vi "claustering trial 1.vi"() -> ()   [LabVIEW 2014]
panel:
  in  "List of common substrings and the number of times they occur":string[][](array[string])
  out "appended array 3":i32[](array[numeric])
  out "appended array 2":i32[](array[numeric])
  out "appended array":dbl[][][](array[numeric])
  in  "milliseconds to wait":u32
  out "3":string[](array[string])
  out "2":string[](array[string])
  out "1":string[](array[string])
  out "0":string[](array[string])
  out "Array":dbl[][](array[numeric])
  out "Weighted arrays 2":dbl[][][](array[numeric])
  out "Weighted arrays of cluster centers":dbl[][][](array[numeric])
  in  "Cluster centers":string[](array[string])=["-2 0 3 0 -3 0 4 -4 0\r\n", "0 3\r\n", "0 4 -3 0 -4 1 0 4 -3 0\r\n", "0\r\n", "-2 0 3 -3 0 -4 1 -4 0 3 -3 4 -3 0 2 0 3\r\n", "0 3 0 1\r\n", "0 1 0 3\r\n", "0 3 -2 0 4\r\n", "0\r\n", "0 -3 4 0 2 -2 0 -3 0 3 -2 3 -3 4\r\n", "0 -3 4 -3 0\r\n", "-2 0 -2 2 0\r\n", "0 3 -2\r\n", "0 4 -3 0 3 -2 0 -3 4 -3 0 3 -2 2 -2 0 4 0\r\n", "2 0 1 -4 0 3 0 -4 4 0 -4 4 0 2 0 4 0 -3 4 -3 0 -4 0 4\r\n", "0 4\r\n", "-2 0 -2 0 3 0\r\n", "0 3 0 -2 3\r\n", "0 4 0 4 -4 0 2 0 -4 4 -3 0 -2 2 -2 0 4 -3 0 2 0 3 0\r\n", "0 4 -3 0 1 -1 0 3 0 -2 2 -2 0 -3 4 -3 0 4 -4 1 0\r\n", "", "0 -3\r\n", "2 0 3 0 1 0 -2 3\r\n", "0\r\n", "1 -1 0\r\n", "0 -2 3 0\r\n", "0 1 0 4 0 4 -4 4\r\n", "0 1 -1 0 3\r\n", "0 2 -2 3 -3 4\r\n", "-2 2 0 -2 3\r\n", "0 -1\r\n", "0 4 -4 4 0 3 0 -2 0 -4 0 1 -4\r\n", "-2 0 4 0 -3 3 0 -2 2 -2 0 -4 0 4 0\r\n", "0 -1 0 -4 4 -4 1 -4 0\r\n", "1 -4 1 0 2 0 -3 0 2 0 -2 0 1 0 1 -4 4 -4 1 0 3 -2 0 -4 4 -4\r\n", "0 1 -4 4 -4 1\r\n", "0 3 0 -3 3 0 1 0 1 -4 4\r\n", "0 1 -4 0 1 -4\r\n", "0 3 -2 0 1 -4 1 0 2 0 4 0 4 0 -1 2 -1 0\r\n", "1 0 -1 0 2 0 4 -4\r\n", "-4\r\n", "-1 0 4\r\n", "0 1 -1 0 1 -4 0\r\n", "-1 0 1 -4 0 3 0 2 0 4 0 -4 4 -4 0 -1 0 -4 0 -2 0 4\r\n", "0 4 0\r\n", "0 4 -4 0 2 -1 0 2 0 4 -4 1 -4 4 0 3\r\n", "0 4 0 2 0\r\n", "1 0 -1 1 0 -4 1 -4 1 0 -4\r\n", "0 3 -2 0 -4\r\n", "2 -1 0 -4 4 -4 0 2 0 4\r\n", "1 0\r\n", "-1 0 -1 1 0 -4\r\n", "0 3 0\r\n", "0 -4 4 -4 0 -4 0 4 0 2 0 1 -4 4\r\n", "-1 0 1 -4\r\n", "-1 0 2 -1 0 2\r\n", "1 -1 0 4 -4 1\r\n", "-1 0 1 -4 4 -4 0 -4 4\r\n", "0 3 0 3 0 1 -1 0 1\r\n", "-1 0 4 0 4 -4 1 0 -4 0\r\n", "1 0 4\r\n", "0 -1 0 2 -1 0 -2 3 -2 0 -4 4 -4\r\n", "0 3 0\r\n", "2 -1 0 1 -4 4 -4 0 2 0\r\n", "0 4 -4 1 0 1 0 1 -4 0 2 0 4 0 4 -4 1\r\n", "1 -1 0 3 0 3 0 1 0 4\r\n", "0 -4 0 -2 0 -4\r\n", "0 -4 4 -4 0 -2 0 2 0\r\n", "-1 0 4 -4 0\r\n", "1 0 -1 2 0 4\r\n", "0 2 0 -2 0\r\n", "0 1 -4 0 -4 0 3 -2 0 -4 0 -4 4 -4 1\r\n", "0 4 0 4 0 4 0 4 0 -2 3 0 3 0 4 0\r\n", "-4 -1\r\n", "-2 0 1 0 -4 4\r\n", "0 4\r\n", "-2 2 0 -1 -4 1 0 3 0\r\n", "-1 0 -1 2\r\n", "0 -1 1 0 4 0 3 -2 0 -2 3 -2 0 4 0 -2 2\r\n", "2 -1 0 4\r\n", "0 4 0 2 0 -2 0\r\n", "1 -1 0 3 0 -4 4 -4 0\r\n", "2 -1 0 3 -2 0 -3 0 3 0 -3 0\r\n", "0 4 0 4 -4 1 -1 0 -3 0 1 -4 1 0 4 0 -4 0 -4 4 -4 1\r\n", "0 -4 1 0 -4 4\r\n", "0 4 0 -2 2 -2 2 -2 2\r\n", "-2 2 -1 0 4 0 2 0 4 0 2 -2 0 4\r\n", "1 0 -1 0 -1 0 1 -1\r\n", "-2 2 -2 3\r\n", "1 0 -1 0 -1 2 0 2 -2 0 -4 0\r\n", "-2 2 0 3 -2 2\r\n", "0\r\n", "1 -1 0 3\r\n", "0 4 0\r\n", "-2 0 1 -4 0 -3 0\r\n", "1 0 -1 2 -1 1 -4\r\n", "0 4\r\n", "-2 0 -1 1\r\n", "0 3 0 3 0 3 -2\r\n", "-4 0 -4 4\r\n", "0 4 0 -4 0 -4\r\n", "-2 2 0 4 -4 0 2 -2\r\n", "-2 2 -2 0 -1\r\n", "0 4 -3 0\r\n", "0 1 0 -1 1\r\n", "-4 0\r\n", "-2 0 3 0 1 0 3 -2 0 -1 0 4 0 3 0 -3 3 -3\r\n", "0 4 0 -2 0 1 0 -4 4 -3 0 1 0 4 0 -4 1 0 3 -3 0\r\n", "0 -1 2\r\n", "2 0 -3 4 0\r\n", "-4 0 -3 3 -3 0 -3 3 0 -2 3 0\r\n", "0 -1 1 -4 4 -3 0 3 0\r\n", "0 -1 2 0 3 0 1 -4 4 0 2 0\r\n", "2 -2 0 -4 0 -4 4 0 -4\r\n", "1 -1 2 -1\r\n", "2 0 -2 0 4 0 2 0 3 0 -2 0 -4\r\n", "1 -1 0 -1\r\n", "0 1 -4 1\r\n", "0 4 0 -1 1 -1 0\r\n", "0 3\r\n", "-2 0\r\n", "1 -4 0 -2 0 4 0 -4 0 4 -3 0 1 -4 0 1\r\n", "0 -3 3 -2 0 3 0 -2 2\r\n", "1 0\r\n", "2\r\n", "0 -4\r\n", "0 4 0 -4 0 -3 3 -3 0 -2 0 -2 0 4 0 -1 1 0 3 0 -4 1 -4 0 4\r\n", "2 0 -1 1\r\n", "0 2 0 4 0 4 -4 0 -1 2\r\n", "0 3 -2 0 3 -2\r\n", "1 0 -3 3 0 -4\r\n", "0 -3 3 0 -1 0\r\n", "2 -2 0 1\r\n", "-4 1 -4 1 -4 0\r\n", "0 4 0 2 0 -4 1 2 -1 0 4 0 1 0 4 -4 4 0 -4 4 0\r\n", "-2 0 3 0 -2 0\r\n"]
  in  "Full transition sequence from service to end":string[](array[string])=["-2 0 3 0 -3 0 4 -4 0\r\n", "0 3\r\n", "0 4 -3 0 -4 1 0 4 -3 0\r\n", "0\r\n", "-2 0 3 -3 0 -4 1 -4 0 3 -3 4 -3 0 2 0 3\r\n", "0 3 0 1\r\n", "0 1 0 3\r\n", "0 3 -2 0 4\r\n", "0\r\n", "0 -3 4 0 2 -2 0 -3 0 3 -2 3 -3 4\r\n", "0 -3 4 -3 0\r\n", "-2 0 -2 2 0\r\n", "0 3 -2\r\n", "0 4 -3 0 3 -2 0 -3 4 -3 0 3 -2 2 -2 0 4 0\r\n", "2 0 1 -4 0 3 0 -4 4 0 -4 4 0 2 0 4 0 -3 4 -3 0 -4 0 4\r\n", "0 4\r\n", "-2 0 -2 0 3 0\r\n", "0 3 0 -2 3\r\n", "0 4 0 4 -4 0 2 0 -4 4 -3 0 -2 2 -2 0 4 -3 0 2 0 3 0\r\n", "0 4 -3 0 1 -1 0 3 0 -2 2 -2 0 -3 4 -3 0 4 -4 1 0\r\n", "", "0 -3\r\n", "2 0 3 0 1 0 -2 3\r\n", "0\r\n", "1 -1 0\r\n", "0 -2 3 0\r\n", "0 1 0 4 0 4 -4 4\r\n", "0 1 -1 0 3\r\n", "0 2 -2 3 -3 4\r\n", "-2 2 0 -2 3\r\n", "0 -1\r\n", "0 4 -4 4 0 3 0 -2 0 -4 0 1 -4\r\n", "-2 0 4 0 -3 3 0 -2 2 -2 0 -4 0 4 0\r\n", "0 -1 0 -4 4 -4 1 -4 0\r\n", "1 -4 1 0 2 0 -3 0 2 0 -2 0 1 0 1 -4 4 -4 1 0 3 -2 0 -4 4 -4\r\n", "0 1 -4 4 -4 1\r\n", "0 3 0 -3 3 0 1 0 1 -4 4\r\n", "0 1 -4 0 1 -4\r\n", "0 3 -2 0 1 -4 1 0 2 0 4 0 4 0 -1 2 -1 0\r\n", "1 0 -1 0 2 0 4 -4\r\n", "-4\r\n", "-1 0 4\r\n", "0 1 -1 0 1 -4 0\r\n", "-1 0 1 -4 0 3 0 2 0 4 0 -4 4 -4 0 -1 0 -4 0 -2 0 4\r\n", "0 4 0\r\n", "0 4 -4 0 2 -1 0 2 0 4 -4 1 -4 4 0 3\r\n", "0 4 0 2 0\r\n", "1 0 -1 1 0 -4 1 -4 1 0 -4\r\n", "0 3 -2 0 -4\r\n", "2 -1 0 -4 4 -4 0 2 0 4\r\n", "1 0\r\n", "-1 0 -1 1 0 -4\r\n", "0 3 0\r\n", "0 -4 4 -4 0 -4 0 4 0 2 0 1 -4 4\r\n", "-1 0 1 -4\r\n", "-1 0 2 -1 0 2\r\n", "1 -1 0 4 -4 1\r\n", "-1 0 1 -4 4 -4 0 -4 4\r\n", "0 3 0 3 0 1 -1 0 1\r\n", "-1 0 4 0 4 -4 1 0 -4 0\r\n", "1 0 4\r\n", "0 -1 0 2 -1 0 -2 3 -2 0 -4 4 -4\r\n", "0 3 0\r\n", "2 -1 0 1 -4 4 -4 0 2 0\r\n", "0 4 -4 1 0 1 0 1 -4 0 2 0 4 0 4 -4 1\r\n", "1 -1 0 3 0 3 0 1 0 4\r\n", "0 -4 0 -2 0 -4\r\n", "0 -4 4 -4 0 -2 0 2 0\r\n", "-1 0 4 -4 0\r\n", "1 0 -1 2 0 4\r\n", "0 2 0 -2 0\r\n", "0 1 -4 0 -4 0 3 -2 0 -4 0 -4 4 -4 1\r\n", "0 4 0 4 0 4 0 4 0 -2 3 0 3 0 4 0\r\n", "-4 -1\r\n", "-2 0 1 0 -4 4\r\n", "0 4\r\n", "-2 2 0 -1 -4 1 0 3 0\r\n", "-1 0 -1 2\r\n", "0 -1 1 0 4 0 3 -2 0 -2 3 -2 0 4 0 -2 2\r\n", "2 -1 0 4\r\n", "0 4 0 2 0 -2 0\r\n", "1 -1 0 3 0 -4 4 -4 0\r\n", "2 -1 0 3 -2 0 -3 0 3 0 -3 0\r\n", "0 4 0 4 -4 1 -1 0 -3 0 1 -4 1 0 4 0 -4 0 -4 4 -4 1\r\n", "0 -4 1 0 -4 4\r\n", "0 4 0 -2 2 -2 2 -2 2\r\n", "-2 2 -1 0 4 0 2 0 4 0 2 -2 0 4\r\n", "1 0 -1 0 -1 0 1 -1\r\n", "-2 2 -2 3\r\n", "1 0 -1 0 -1 2 0 2 -2 0 -4 0\r\n", "-2 2 0 3 -2 2\r\n", "0\r\n", "1 -1 0 3\r\n", "0 4 0\r\n", "-2 0 1 -4 0 -3 0\r\n", "1 0 -1 2 -1 1 -4\r\n", "0 4\r\n", "-2 0 -1 1\r\n", "0 3 0 3 0 3 -2\r\n", "-4 0 -4 4\r\n", "0 4 0 -4 0 -4\r\n", "-2 2 0 4 -4 0 2 -2\r\n", "-2 2 -2 0 -1\r\n", "0 4 -3 0\r\n", "0 1 0 -1 1\r\n", "-4 0\r\n", "-2 0 3 0 1 0 3 -2 0 -1 0 4 0 3 0 -3 3 -3\r\n", "0 4 0 -2 0 1 0 -4 4 -3 0 1 0 4 0 -4 1 0 3 -3 0\r\n", "0 -1 2\r\n", "2 0 -3 4 0\r\n", "-4 0 -3 3 -3 0 -3 3 0 -2 3 0\r\n", "0 -1 1 -4 4 -3 0 3 0\r\n", "0 -1 2 0 3 0 1 -4 4 0 2 0\r\n", "2 -2 0 -4 0 -4 4 0 -4\r\n", "1 -1 2 -1\r\n", "2 0 -2 0 4 0 2 0 3 0 -2 0 -4\r\n", "1 -1 0 -1\r\n", "0 1 -4 1\r\n", "0 4 0 -1 1 -1 0\r\n", "0 3\r\n", "-2 0\r\n", "1 -4 0 -2 0 4 0 -4 0 4 -3 0 1 -4 0 1\r\n", "0 -3 3 -2 0 3 0 -2 2\r\n", "1 0\r\n", "2\r\n", "0 -4\r\n", "0 4 0 -4 0 -3 3 -3 0 -2 0 -2 0 4 0 -1 1 0 3 0 -4 1 -4 0 4\r\n", "2 0 -1 1\r\n", "0 2 0 4 0 4 -4 0 -1 2\r\n", "0 3 -2 0 3 -2\r\n", "1 0 -3 3 0 -4\r\n", "0 -3 3 0 -1 0\r\n", "2 -2 0 1\r\n", "-4 1 -4 1 -4 0\r\n", "0 4 0 2 0 -4 1 2 -1 0 4 0 1 0 4 -4 4 0 -4 4 0\r\n", "-2 0 3 0 -2 0\r\n"]
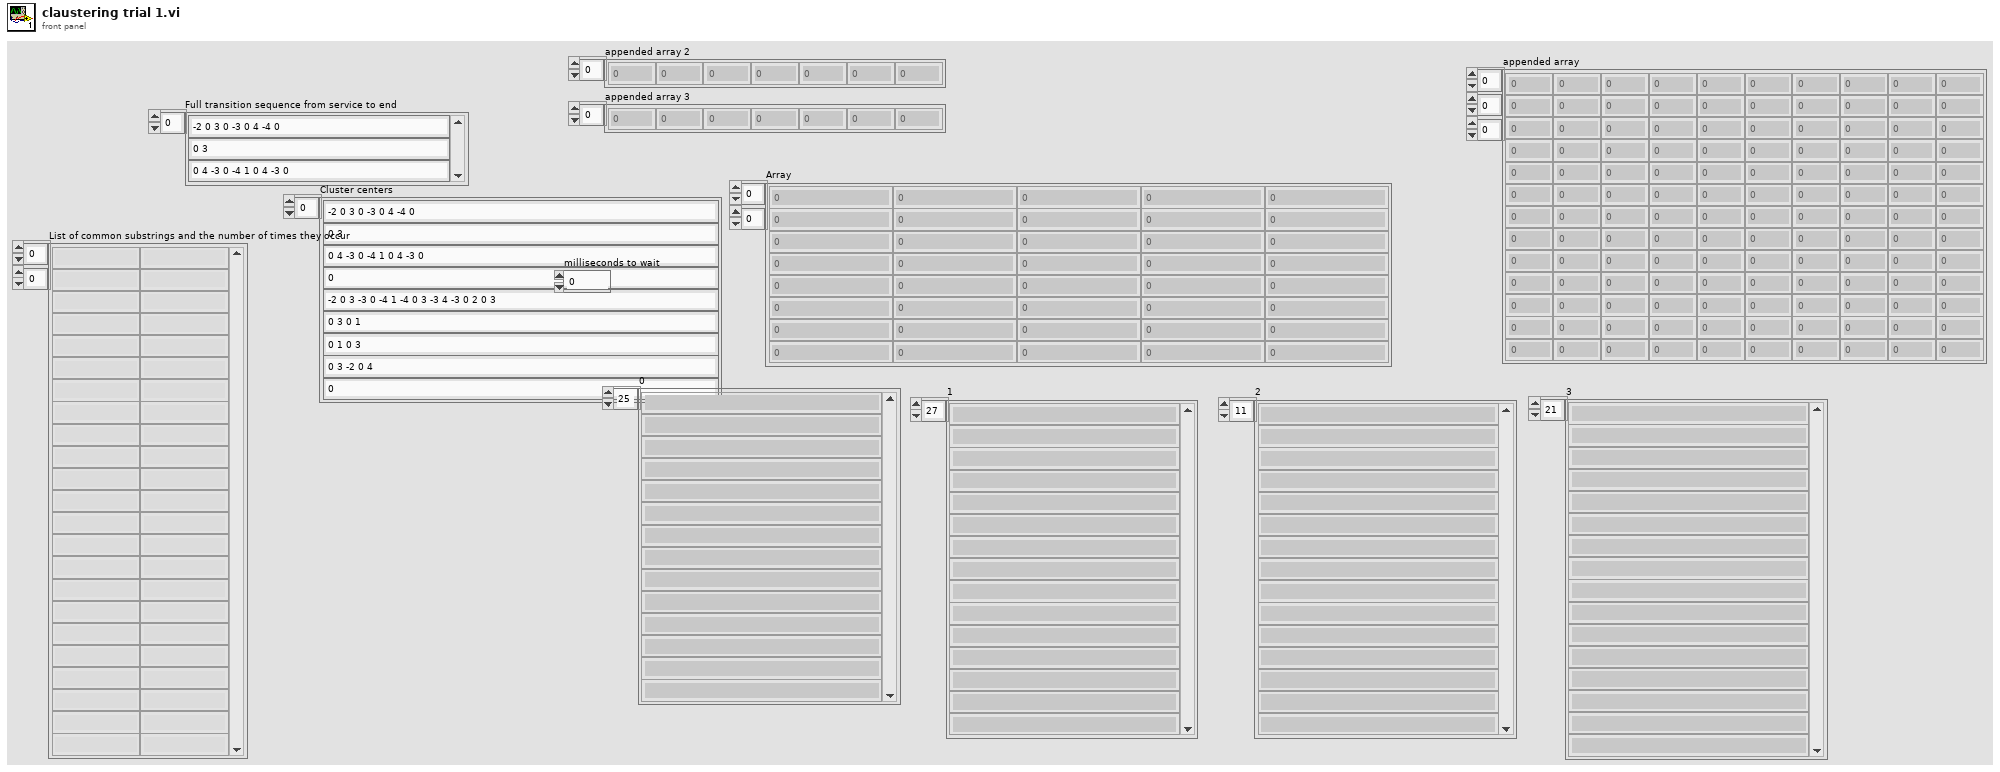
[diagram p1: front panel]
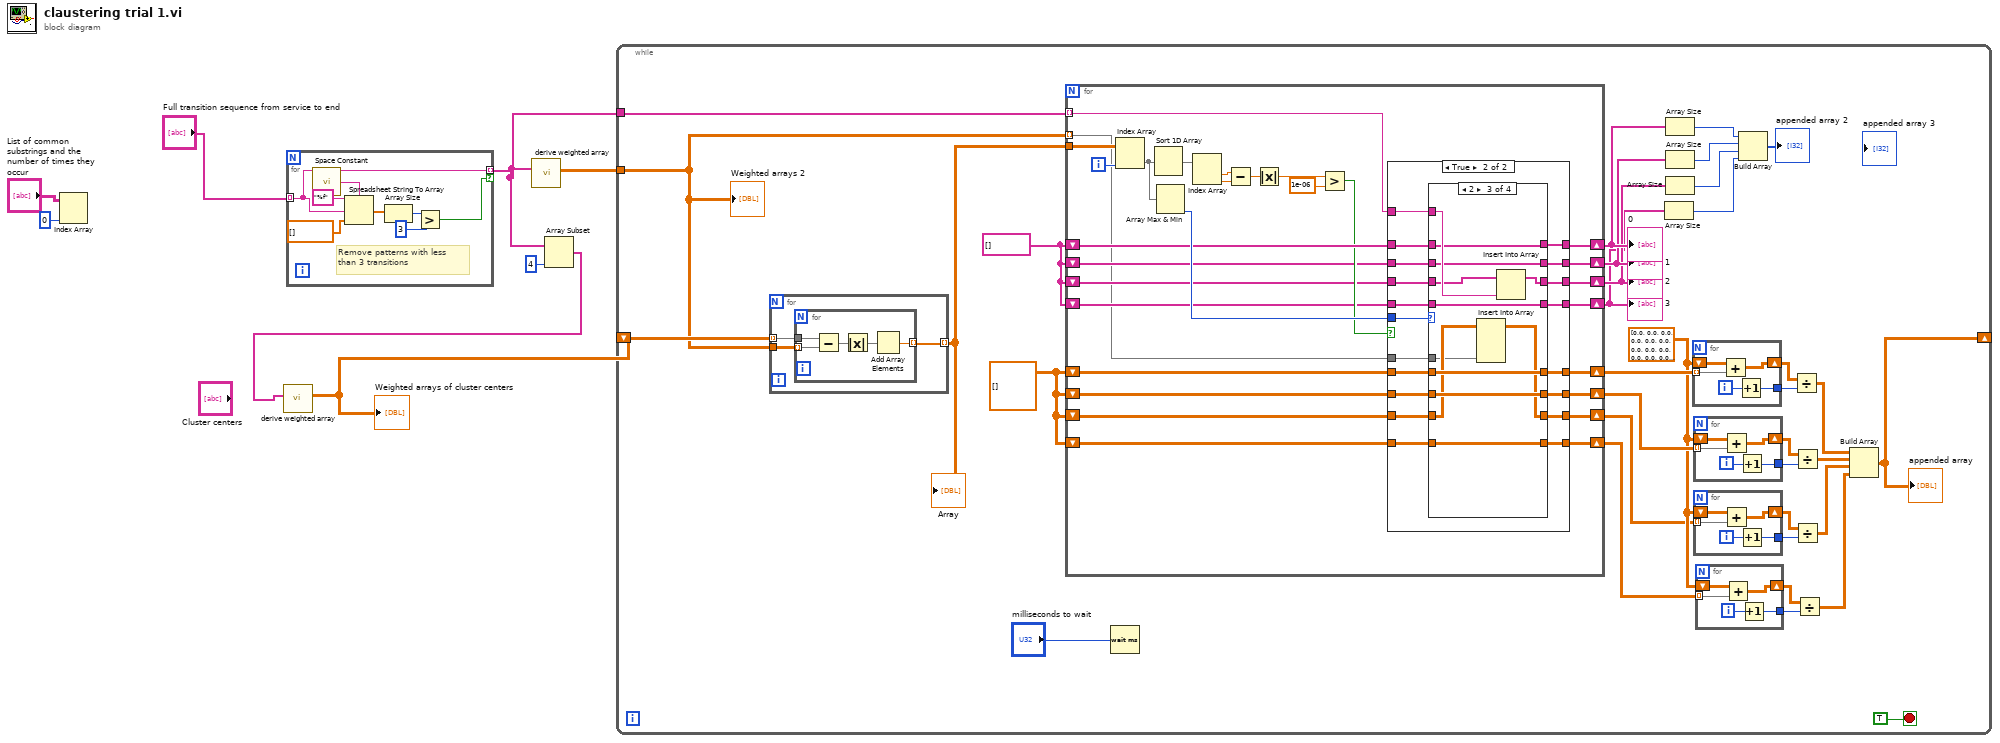
[diagram p0: block diagram]
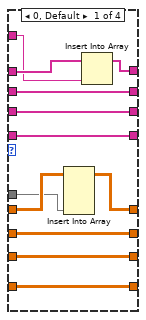
[diagram p3: hidden frame]
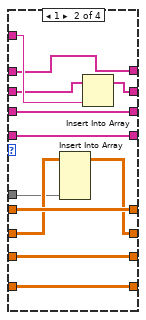
[diagram p4: hidden frame]
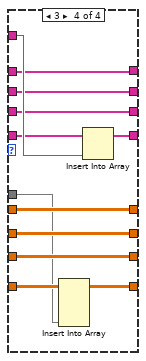
[diagram p5: hidden frame]
diagram:
  n1 = Index Array(array="List of common substrings and the number of times they occur", index (col)=0 ("disabled index (col)")) -> ()  [unwired: 1 in, 1 out]
  n2 = for {
    tunnel: "Full transition sequence from service to end" -> [w10] mode=indexing
    tunnel: [w10] -> w4 mode=indexing if=w9
    # "Remove patterns with less \nthan 3 transitions"
    n3 = call <vilib>:"Space Constant.vi"() -> ("String"=w15:string)
    n4 = Spreadsheet String To Array(delimiter (Tab)=w15, format string="%f", spreadsheet string=w10, array type (2D Dbl)=dbl[] [] ("array 2")) -> (array=w13:dbl[])
    n5 = Array Size(array=w13) -> (size(s)=w12:i32)
    n6 = Greater?(x=w12, y=3) -> (0:w9:bool)
  }
  n7 = call "derive weighted array.vi"("Full transition sequence from service to end"=w4) -> ("Weighted arrays"=w1:dbl[][][])  [unwired: 10 in]
  n8 = Array Subset(array=w4, length=4) -> (w3:string[])  [unwired: 1 in]
  n9 = call "derive weighted array.vi"("Full transition sequence from service to end"=w3) -> ("Weighted arrays"=w2:dbl[][][])  [unwired: 10 in]
  "Weighted arrays of cluster centers" <- w2
  n10 = while {
    tunnel: w4 -> [w49]
    shift-right: [w26] -> _
    shift-left: w2 -> [w51]
    tunnel: w1 -> [w50]
    stop <- TRUE stop-if-true
    w35 = dbl[][] [[0.0, 0.0, 0.0, 0.0, 0.0], [0.0, 0.0, 0.0, 0.0, 0.0], [0.0, 0.0, 0.0, 0.0, 0.0], [0.0, 0.0, 0.0, 0.0, 0.0], [0.0, 0.0, 0.0, 0.0, 0.0]] ("Weighted arrays")
    w46 = dbl[][][] [] ("Weighted arrays")
    w47 = string[] [] ("Full transition sequence from service to end")
    n11 = for {
      tunnel: w51 -> [w178] mode=indexing
      tunnel: w50 -> [w177]
      tunnel: [w176] -> w48 mode=indexing
      n12 = for {
        tunnel: w178 -> [w183]
        tunnel: w177 -> [w182] mode=indexing
        tunnel: [w179] -> w176 mode=indexing
        n13 = Subtract(x=w183, y=w182) -> (x-y=w181:dbl[][])
        n14 = Absolute Value(x=w181) -> (abs(x)=w180:dbl[][])
        n15 = Add Array Elements(numeric array=w180) -> (sum=w179:dbl)
      }
    }
    "Array" <- w48
    n16 = for {
      tunnel: w49 -> [w89] mode=indexing
      tunnel: w50 -> [w80] mode=indexing
      tunnel: w48 -> [w100]
      shift-right: [w88] -> w25
      shift-left: w47 -> [w90]
      shift-right: [w86] -> w24
      shift-left: w47 -> [w83]
      shift-right: [w85] -> w23
      shift-left: w47 -> [w82]
      shift-right: [w84] -> w22
      shift-left: w47 -> [w81]
      shift-right: [w79] -> w45
      shift-left: w46 -> [w78]
      shift-right: [w74] -> w36
      shift-left: w46 -> [w77]
      shift-right: [w73] -> w34
      shift-left: w46 -> [w76]
      shift-right: [w72] -> w33
      shift-left: w46 -> [w75]
      i -> [w93]
      n17 = Index Array(array=w100, index (col)=w93) -> (element=w92:dbl[])  [unwired: 1 in]
      n18 = Sort 1D Array(array=w92) -> (sorted array=w95:dbl[])
      n19 = Array Max & Min(array=w92) -> (min index (indices)=w91:i32)  [unwired: 3 out]
      n20 = Index Array(array=w95) -> (element #1=w99:dbl, element #2=w94:dbl)  [unwired: 2 in]
      n21 = Subtract(x=w99, y=w94) -> (x-y=w97:dbl)
      n22 = Absolute Value(x=w97) -> (abs(x)=w96:dbl)
      n23 = Greater?(x=w96, y=1e-06) -> (0:w87:bool)
      n24 = case shown="True" w87 {
        tunnel: w91 -> [_ w127]
        tunnel: w90 -> [w108 w126]
        tunnel: w89 -> [_ w125]
        tunnel: [w108 w124] -> w88
        tunnel: [w107 w120] -> w86
        tunnel: [w106 w119] -> w85
        tunnel: [w105 w118] -> w84
        tunnel: w83 -> [w107 w123]
        tunnel: w82 -> [w106 w122]
        tunnel: w81 -> [w105 w121]
        tunnel: w80 -> [_ w117]
        tunnel: [w104 w115] -> w79
        tunnel: w78 -> [w104 w116]
        tunnel: w77 -> [w103 w114]
        tunnel: w76 -> [w102 w113]
        tunnel: w75 -> [w101 w112]
        tunnel: [w103 w111] -> w74
        tunnel: [w102 w110] -> w73
        tunnel: [w101 w109] -> w72
        frame False {
        }
        frame True {
          n25 = case shown="2" w127 {
            tunnel: w126 -> [w139 w146 w161 w174]
            tunnel: w125 -> [w138 w151 w163 w175]
            tunnel: [w137 w146 w161 w174] -> w124
            tunnel: w123 -> [w136 w147 w158 w173]
            tunnel: w122 -> [w135 w150 w159 w170]
            tunnel: w121 -> [w134 w149 w162 w171]
            tunnel: [w136 w148 w158 w173] -> w120
            tunnel: [w135 w150 w160 w170] -> w119
            tunnel: [w134 w149 w162 w172] -> w118
            tunnel: w117 -> [w132 w141 w153 w165]
            tunnel: w116 -> [w133 w145 w157 w169]
            tunnel: [w131 w145 w157 w169] -> w115
            tunnel: w114 -> [w130 w142 w156 w168]
            tunnel: w113 -> [w129 w144 w154 w167]
            tunnel: w112 -> [w128 w143 w155 w166]
            tunnel: [w130 w140 w156 w168] -> w111
            tunnel: [w129 w144 w152 w167] -> w110
            tunnel: [w128 w143 w155 w164] -> w109
            frame 0, Default {
              n26 = Insert Into Array(array=w133, new element=w132) -> (w131:dbl[][][])  [unwired: 3 in]
              n27 = Insert Into Array(array=w139, new element=w138) -> (w137:string[])  [unwired: 1 in]
            }
            frame 1 {
              n28 = Insert Into Array(array=w142, new element=w141) -> (w140:dbl[][][])  [unwired: 3 in]
              n29 = Insert Into Array(array=w147, new element=w151) -> (w148:string[])  [unwired: 1 in]
            }
            frame 2 {
              n30 = Insert Into Array(array=w154, new element=w153) -> (w152:dbl[][][])  [unwired: 3 in]
              n31 = Insert Into Array(array=w159, new element=w163) -> (w160:string[])  [unwired: 1 in]
            }
            frame 3 {
              n32 = Insert Into Array(array=w166, new element=w165) -> (w164:dbl[][][])  [unwired: 3 in]
              n33 = Insert Into Array(array=w171, new element=w175) -> (w172:string[])  [unwired: 1 in]
            }
          }
        }
      }
    }
    "0" <- w25
    "1" <- w24
    "2" <- w23
    "3" <- w22
    n34 = Wait (ms)(milliseconds to wait="milliseconds to wait") -> ()  [unwired: 1 out]
    n35 = Array Size(array=w22) -> (size(s)=w18:i32)
    n36 = Array Size(array=w25) -> (size(s)=w21:i32)
    n37 = Array Size(array=w24) -> (size(s)=w20:i32)
    n38 = Array Size(array=w23) -> (size(s)=w19:i32)
    n39 = for {
      tunnel: w45 -> [w70] mode=indexing
      shift-right: [w69] -> w44
      shift-left: w35 -> [w71]
      tunnel: [w67] -> w43
      i -> [w68]
      n40 = Add(x=w71, y=w70) -> (x+y=w69:dbl[][])
      n41 = Increment(x=w68) -> (x+1=w67:i32)
    }
    n42 = for {
      tunnel: w36 -> [w65] mode=indexing
      shift-right: [w64] -> w41
      shift-left: w35 -> [w66]
      tunnel: [w62] -> w42
      i -> [w63]
      n43 = Add(x=w66, y=w65) -> (x+y=w64:dbl[][])
      n44 = Increment(x=w63) -> (x+1=w62:i32)
    }
    n45 = for {
      tunnel: w34 -> [w60] mode=indexing
      shift-right: [w59] -> w40
      shift-left: w35 -> [w61]
      tunnel: [w57] -> w39
      i -> [w58]
      n46 = Add(x=w61, y=w60) -> (x+y=w59:dbl[][])
      n47 = Increment(x=w58) -> (x+1=w57:i32)
    }
    n48 = for {
      tunnel: w33 -> [w55] mode=indexing
      shift-right: [w54] -> w37
      shift-left: w35 -> [w56]
      tunnel: [w52] -> w38
      i -> [w53]
      n49 = Add(x=w56, y=w55) -> (x+y=w54:dbl[][])
      n50 = Increment(x=w53) -> (x+1=w52:i32)
    }
    n51 = Build Array(w21, w20, w19, w18) -> (→"appended array 2":i32[])
    n52 = Divide(x=w44, y=w43) -> (x/y=w32:dbl[][])
    n53 = Divide(x=w41, y=w42) -> (x/y=w31:dbl[][])
    n54 = Divide(x=w40, y=w39) -> (x/y=w30:dbl[][])
    n55 = Divide(x=w37, y=w38) -> (x/y=w29:dbl[][])
    n56 = Build Array(w32, w31, w30, w29) -> (w26:dbl[][][])
    "appended array" <- w26
    "Weighted arrays 2" <- w50
  }
